vi "GetSubset.vi"(9 "omega":dbl, 10 "FFT":cdb[](array[numeric]), 11 "mag":cluster{i32, dbl, dbl[]}(graph)={0, 0.006283248139660982, array[25000 elements]}) -> (0 "r":dbl format="%.6f", 1 "w_r":dbl, 2 "mag 2":cluster{dbl[], dbl[]}(graph), 3 "Niquist":cluster{dbl[], dbl[]}[](graph), 5 "angle":cluster{dbl[], "yi":dbl[]}[](graph))   [LabVIEW 2022 SP3]
uses:
  <vilib>/gmath/NI_Gmath.lvlib
  <vilib>/Analysis/NI_AALPro.lvlib
panel:
  in  "OK Button":bool
  out "derivative":cluster{dbl[], "Best Polynomial Fit":dbl[]}[](graph)
  in  "polynomial order":i32=2
  out "Polynomial Coefficients":dbl[](array[numeric])
  out "mag 2":cluster{i32, dbl, dbl[]}(graph)
  in  "y":i32=5
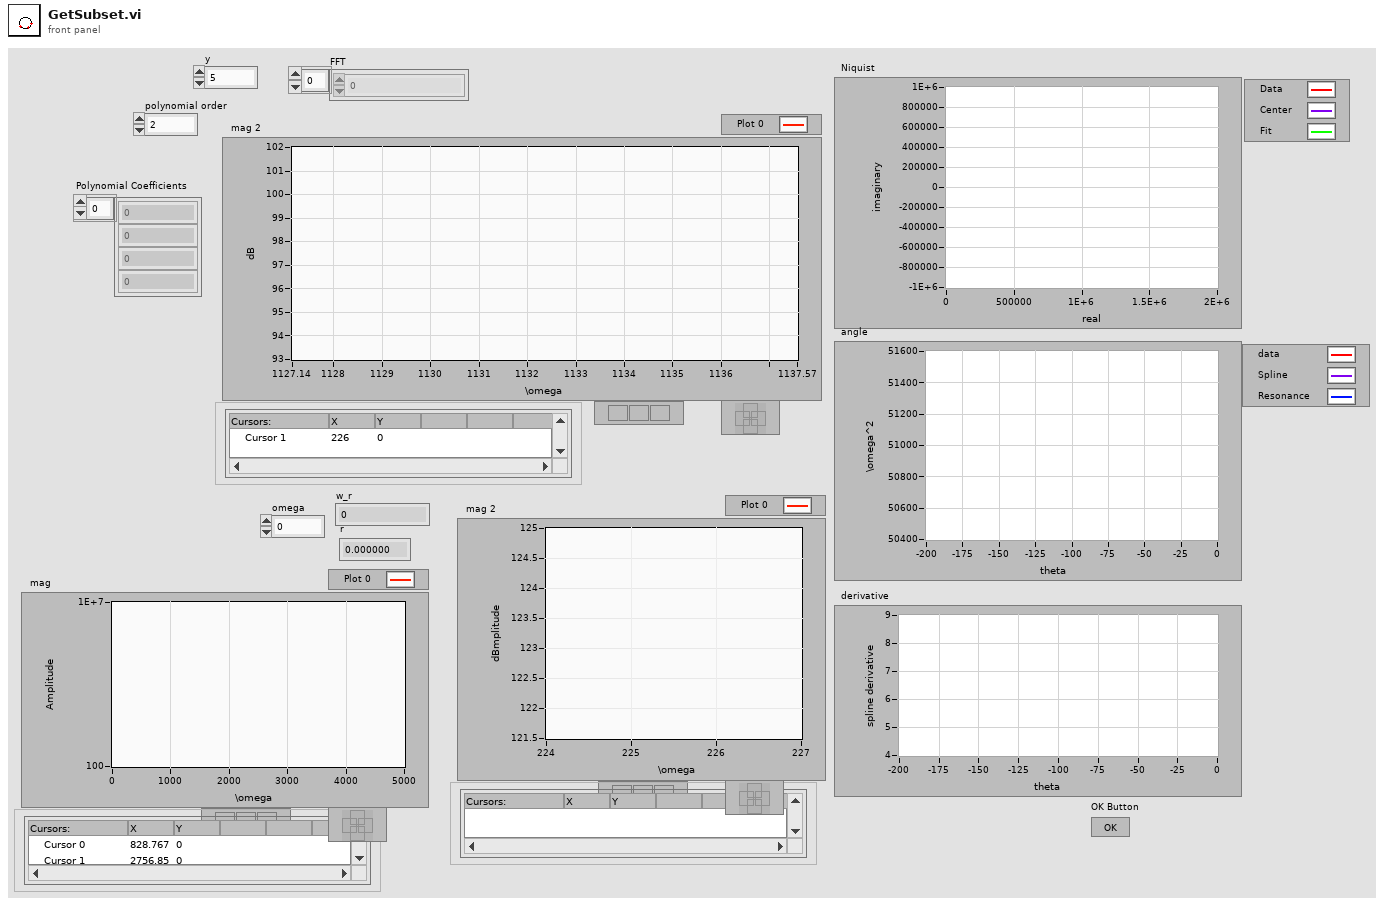
[diagram p1: front panel]
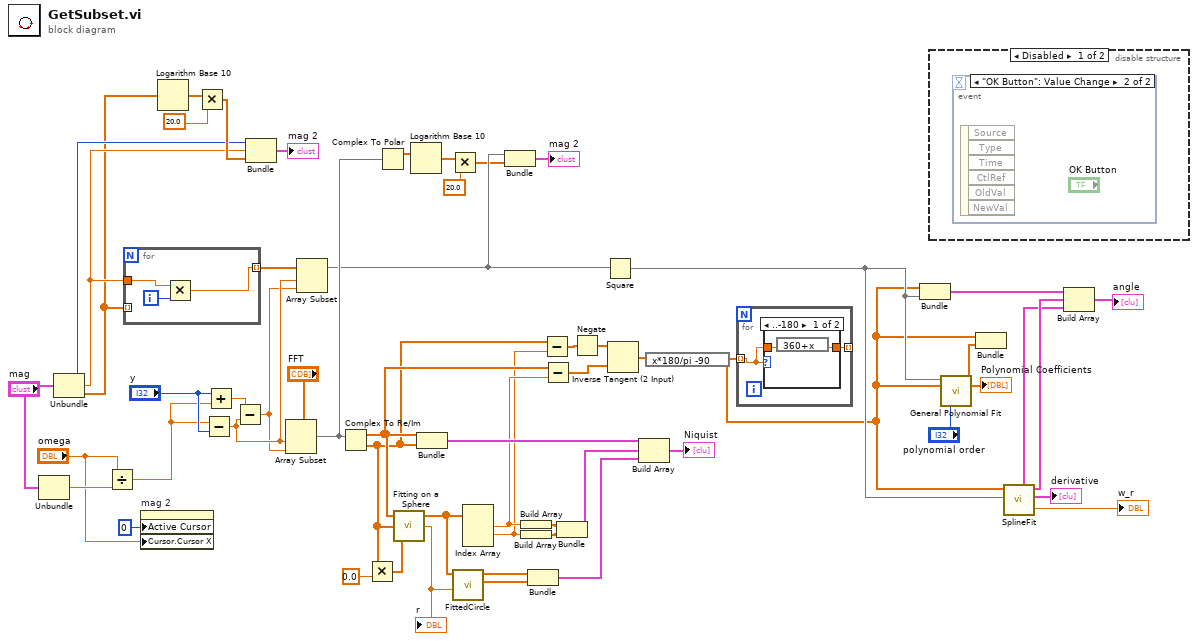
[diagram p0: block diagram]
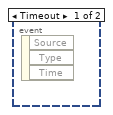
[diagram p2: hidden frame]
diagram:
  n1 = Unbundle("mag") -> (w20:dbl)  [unwired: 2 out]
  n2 = Unbundle("mag") -> (w18:i32, w4:dbl, w3:dbl[])
  n3 = Divide(x="omega", y=w20) -> (x/y=w19:dbl)
  n4 = for {
    tunnel: w4 -> [w58]
    tunnel: w3 -> [_] mode=indexing
    tunnel: [w57] -> w39 mode=indexing
    i -> [w59]
    n5 = Multiply(x=w58, y=w59) -> (x*y=w57:dbl)
  }
  n6 = property on="mag 2" class="WFGraph (strict)"("Active Cursor"=u32 0, "Cursor.Cursor X"="omega") -> ()  [unwired: 2 in, 2 out]
  n7 = Logarithm Base 10(1:w3) -> (0:w35:dbl[])
  n8 = Multiply(x=20.0, y=w35) -> (x*y=w33:dbl[])
  n9 = Subtract(x=w19, y="y") -> (x-y=w28:dbl)
  n10 = Add(x="y", y=w19) -> (x+y=w54:dbl)
  n11 = Subtract(x=w54, y=w28) -> (x-y=w27:dbl)
  n12 = Bundle(w18, w4, w33) -> (→"mag 2":cluster{i32, dbl, dbl[]})  [unwired: 1 in]
  n13 = Array Subset(array="FFT", index=w28, length=w27) -> (w17:cdb[])
  n14 = Array Subset(array=w39, index=w28, length=w27) -> (w16:dbl[])
  n15 = Complex To Re/Im(x + iy=w17) -> (x=w42:dbl[], y=w37:dbl[])
  n16 = Multiply(x=w37, y=0.0) -> (x*y=w48:dbl[])
  n17 = Complex To Polar(r * e^(i*theta)=w17) -> (r=w6:dbl[])  [unwired: 1 out]
  n18 = call <vilib>:"Fitting on a Sphere.vi"("Z"=w48, "Y"=w37, "X"=w42) -> ("r"=w46:dbl, "x0, y0, z0"=w43:dbl[])  [unwired: 1 out]
  "r" <- w46
  n19 = Logarithm Base 10(1:w6) -> (0:w9:dbl[])
  n20 = Bundle(w42, w37) -> (w55:cluster{dbl[], dbl[]})  [unwired: 1 in]
  n21 = Multiply(x=20.0, y=w9) -> (x*y=w7:dbl[])
  n22 = call "FittedCircle.vi"("r"=w46, "x0, y0, z0"=w43) -> ("Y"=w45:dbl[], "X"=w44:dbl[])  [unwired: 8 in]
  n23 = Index Array(array=w43) -> (element #1=w41:dbl, element #2=w36:dbl)  [unwired: 3 in, 1 out]
  n24 = Bundle(w16, w7) -> (→"mag 2":cluster{dbl[], dbl[]})  [unwired: 1 in]
  n25 = Build Array(w41) -> (w51:dbl[])
  n26 = Build Array(w36) -> (w50:dbl[])
  n27 = Bundle("X"=w44, "Y"=w45) -> (w47:cluster{"X":dbl[], "Y":dbl[]})  [unwired: 1 in]
  n28 = Subtract(x=w37, y=w36) -> (x-y=w15:dbl[])
  n29 = Subtract(x=w42, y=w41) -> (x-y=w40:dbl[])
  n30 = Bundle(w51, w50) -> (w52:cluster{dbl[], dbl[]})  [unwired: 1 in]
  n31 = Negate(x=w15) -> (-x=w14:dbl[])
  n32 = Square(x=w16) -> (x^2=w26:dbl[])
  n33 = Inverse Tangent (2 Input)(1:w40, 2:w14) -> (0:w38:dbl[])
  n34 = Build Array(w55, w52, w47) -> (→"Niquist":cluster{"X":dbl[], "Y":dbl[]}[])
  n35 = expression code="x*180/pi -90"(w38) -> (w12:dbl[])
  n36 = for {
    tunnel: w12 -> [w60] mode=indexing
    tunnel: [w61] -> _ mode=indexing
    n37 = case shown="..-180" w60 {
      tunnel: [w62 w64] -> w61
      tunnel: w60 -> [w63 w64]
      frame ..-180 {
        n38 = expression code="360+x"(w63) -> (w62:dbl)
      }
      frame -179.. {
      }
    }
  }
  n39 = Bundle(w12, w26) -> (w13:cluster{dbl[], dbl[]})  [unwired: 1 in]
  n40 = disable-structure shown="Disabled" {
    frame Disabled {
      n41 = event shown="[1] \"OK Button\": Value Change" {
        selector: _ -> [_ _]
        dyn-events: _ -> [_ _]
        timeout: _ -> [_ _]
        event Timeout {
          n42 = event-data() -> ()  [unwired: 1 in, 3 out]
        }
        event "OK Button": Value Change {
          n43 = event-data() -> ()  [unwired: 1 in, 6 out]
        }
      }
    }
    frame Enabled {
    }
  }
  n44 = call <vilib>:"General Polynomial Fit.vi"("Y"=w26, "polynomial order"="polynomial order", "X"=w12) -> ("Best Polynomial Fit"=w30:dbl[], "Polynomial Coefficients"=→"Polynomial Coefficients":dbl[])  [unwired: 9 in, 2 out]
  n45 = Bundle(w12, "Best Polynomial Fit"=w30) -> ()  [unwired: 1 in, 1 out]
  n46 = call "SplineFit.vi"("Y array"=w26, "X array"=w12) -> ("derivative"=→"derivative":cluster{dbl[], "Best Polynomial Fit":dbl[]}[], "Spline"=w25:cluster{dbl[], "dX/dt":dbl[]}, "w_r"=→"w_r":dbl, "Point"=w22:cluster{dbl[], dbl[]})  [unwired: 6 in]
  n47 = Build Array(w13, w25, w22) -> (→"angle":cluster{dbl[], "dX/dt":dbl[]}[])
